vi "Student t PDF.vi"(10 "k degrees of freedom":i32=1, 11 "x":dbl=1.0) -> (0 "error":i32, 3 "pdf(x)":dbl=0.15915494309189535)   [LabVIEW 2020, in "NI_Gmath.lvlib"]
doc: "Computes the continuous probability density function (PDF) of various distributions. You must manually select the polymorphic instance to use."
uses:
  <vilib>/gmath/NI_Gmath.lvlib
  <vilib>/gmath/statdist.llb/st_error_code.ctl
  <vilib>/gmath/SpecialFunctions.llb/Gamma Function.vi
panel:
  # "Student t PDF"
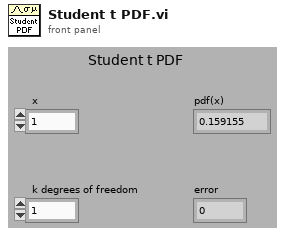
[diagram p1: front panel]
types:
  T1 = typedef "NI_Gmath.lvlib/st_error_code.ctl" = i32
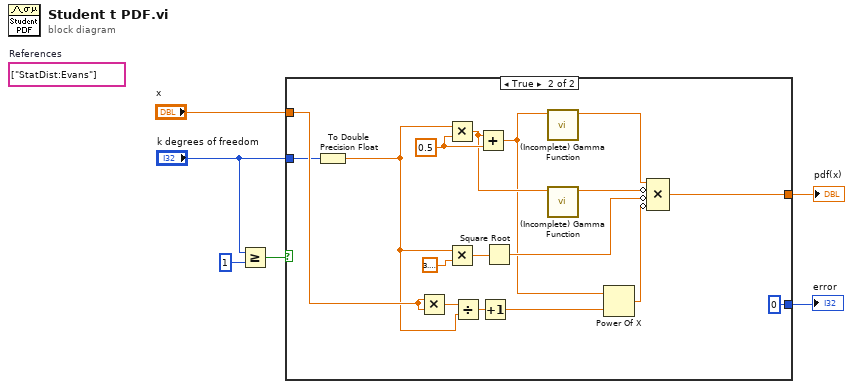
[diagram p0: block diagram]
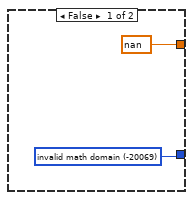
[diagram p2: hidden frame]
diagram:
  (unwired) string[] ["StatDist:Evans"]  # References
  n1 = Greater Or Equal?(x="k degrees of freedom", y=1) -> (x >= y?=w1:bool)
  n2 = case shown="True" w1 {
    tunnel: [w7 0 ("invalid math domain")] -> w6
    tunnel: [nan w24] -> w5
    tunnel: "x" -> [_ w12]
    tunnel: "k degrees of freedom" -> [_ w11]
    frame False {
      w7 = T1 -20069 items=["invalid math domain"=-20069, "Fourier interpolation size m >= n"=-20070, "empty array"=-20003] ("stat interp error code")
    }
    frame True {
      w23 = 0.5 ("x")
      n3 = To Double Precision Float(number=w11) -> (double precision float=w9:dbl)
      n4 = Multiply(x=w12, y=w12) -> (x*y=w16:dbl)
      n5 = Multiply(x=w9, y=w23) -> (x*y=w20:dbl)
      n6 = Multiply(x=w9, y=3.141592653589793) -> (x*y=w17:dbl)
      n7 = Divide(x=w16, y=w9) -> (x/y=w15:dbl)
      n8 = Add(x=w20, y=w23) -> (x+y=w10:dbl)
      n9 = Increment(x=w15) -> (x+1=w14:dbl)
      n10 = Square Root(x=w17) -> (sqrt(x)=w18:dbl)
      n11 = call-poly <vilib>:"(Incomplete) Gamma Function.vi"("x"=w10) -> ("g(x)"=w21:dbl)  [unwired: 10 in]
      n12 = call-poly <vilib>:"(Incomplete) Gamma Function.vi"("x"=w20) -> ("g(x)"=w19:dbl)  [unwired: 10 in]
      n13 = Power Of X(1:w14, 2:w10) -> (0:w13:dbl)
      n14 = Compound Arithmetic op=MULTIPLY(w21, invert w19, invert w18, invert w13) -> (w24:dbl)
    }
  }
  "pdf(x)" <- w5
  "error" <- w6
